vi "Home Axis.vi"(8 "error in (no error)":errorcluster, 11 "FINE SIM Motion Axis":refnum<class "FINE SIM Motion Axis.lvclass">) -> (0 "error out":errorcluster, 3 "FINE SIM Motion Axis":refnum<class "FINE SIM Motion Axis.lvclass">)   [LabVIEW 2022 SP3, in "FINE SIM Motion Axis.lvclass"]
uses:
  FINE SIM Motion Axis.lvclass
  TypeDefs/Homing Status.ctl
  FINE SIM Motion Axis.lvclass/FINE SIM Motion Axis.ctl
  Accessors/Read Sim Axis Data.vi
  Accessors/Write Sim Axis Data.vi
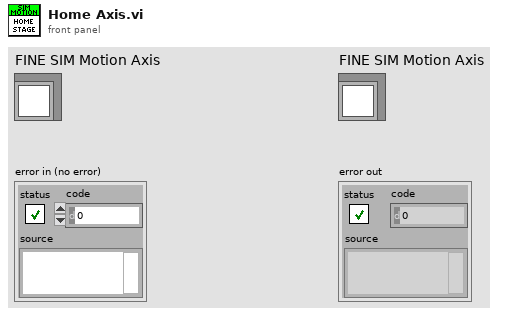
[diagram p1: front panel]
types:
  T1 = typedef "FINE SIM Motion Axis.lvclass/Homing Status.ctl" = enum16{"Idle", "Inital Home Motion", "Final Home Motion", "Done Homing"}
  T2 = typedef "FINE SIM Motion Axis.lvclass/Axis Data.ctl" = cluster{"Axis Parameters":T3, "Axis Settings":T4, "Time Stamp":timestamp}
  T3 = typedef "FINE SIM Motion Axis.lvclass/Axis Parameters.ctl" = cluster{"Moving":bool, "Homed":bool, "Desired Position":dbl, "Current Positon":dbl, "Current Speed":dbl, "Home Status":T1}
  T4 = typedef "FINE SIM Motion Axis.lvclass/Axis Settings.ctl" = cluster{"Speed":dbl, "Acceleration":dbl}
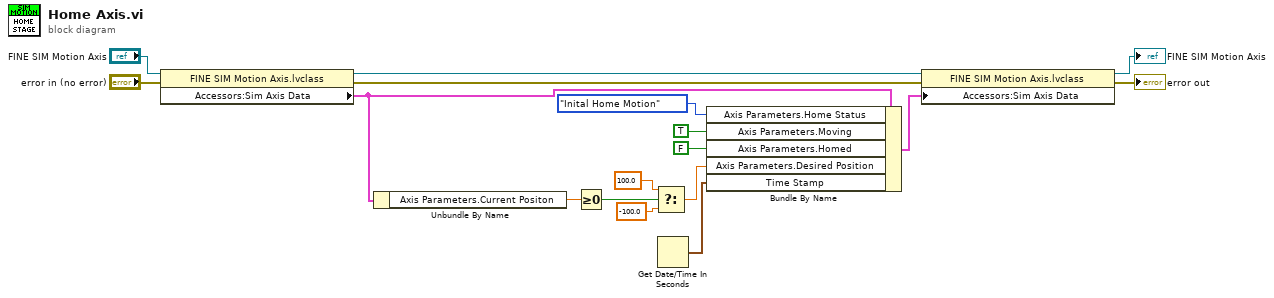
[diagram p0: block diagram]
diagram:
  n1 = property class="FINE SIM Motion Axis.lvclass"(reference="FINE SIM Motion Axis", error in="error in (no error)") -> (reference out=w17:refnum<class "FINE SIM Motion Axis.lvclass">, error out=w6:errorcluster, "Accessors:Sim Axis Data"=w14:T2)
  n2 = Unbundle By Name(w14) -> ("Axis Parameters.Current Positon"=w16:dbl)
  n3 = Greater Or Equal To 0?(x=w16) -> (x >= 0?=w15:bool)
  n4 = Select(t=100.0, s=w15, f=-100.0) -> (s? t:f=w9:dbl)
  n5 = Get Date/Time In Seconds() -> (seconds since 1Jan1904=w3:timestamp)
  n6 = Bundle By Name(cluster=w14, "Axis Parameters.Home Status"=Homing_Status."Inital Home Motion", "Axis Parameters.Moving"=TRUE, "Axis Parameters.Homed"=FALSE, "Axis Parameters.Desired Position"=w9, "Time Stamp"=w3) -> (w8:T2)
  n7 = property class="FINE SIM Motion Axis.lvclass"(reference=w17, error in=w6, "Accessors:Sim Axis Data"=w8) -> (reference out=→"FINE SIM Motion Axis":refnum<class "FINE SIM Motion Axis.lvclass">, error out=→"error out":errorcluster)
